vi "create.vi"(11 "messenger":refnum<class "Send.lvclass">) -> (3 "messenger reporter":refnum<class "messenger reporter.lvclass">)   [LabVIEW 2013, in "messenger reporter.lvclass"]
uses:
  messenger reporter.lvclass
  <vilib>/drjdpowell/Messenging/Core Messengers/Send/Send.lvclass
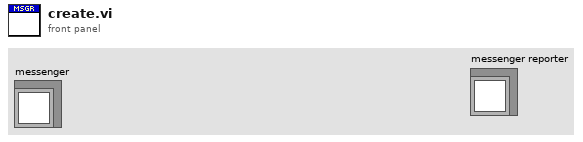
[diagram p1: front panel]
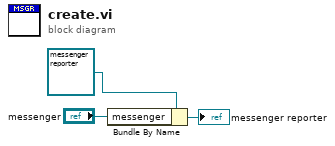
[diagram p0: block diagram]
diagram:
  n1 = Bundle By Name(cluster=refnum<class "messenger reporter.lvclass"> refnum ("messenger reporter in"), "messenger"="messenger") -> (→"messenger reporter":refnum<class "messenger reporter.lvclass">)
